vi "PXI_Host_FXP_Read_OldMethod_Benchmark.vi"() -> ()   [LabVIEW 2018]
uses:
  <vilib>/addons/FPGA Advanced Session Resources/LVFPGA Adv Session Resources/OpenByNameSubVI.vi
  <vilib>/rvi/interface/common/dynamic/niFpgaEscapeDelimiterAndNull.vi
  <vilib>/Utility/error.llb/Error Cluster From Error Code.vi
  <vilib>/rvi/errors/niLvFpgaAdjustHostInterfaceError.vi
  <vilib>/FPGAPlugInAG/Dynamic/niLvFpga_Close_Dynamic.vi
  <vilib>/addons/FPGA Advanced Session Resources/LVFPGA Adv Session Resources/OpenByName.xnode
  <vilib>/rvi/interface/nirviReadWriteControl/nirviReadWriteControl.xnode
  <vilib>/rvi/interface/nirviCloseFPGA/nirviCloseFPGA.xnode
  <vilib>/rvi/interface/Simulation/niFpgaSimulationCallBeginRW.vi
  NiFpgaLv.dll
  <vilib>/addons/FPGA Advanced Session Resources/LVFPGA Adv Session Resources/LVFPGAAdvSessionResources.lvlib
panel:
  out "Value out":fxp<+/-,32,16>
  out "error out":errorcluster
  out "Execution time (s)":dbl
  # "Recorded time"
  # "3.37551E-5"
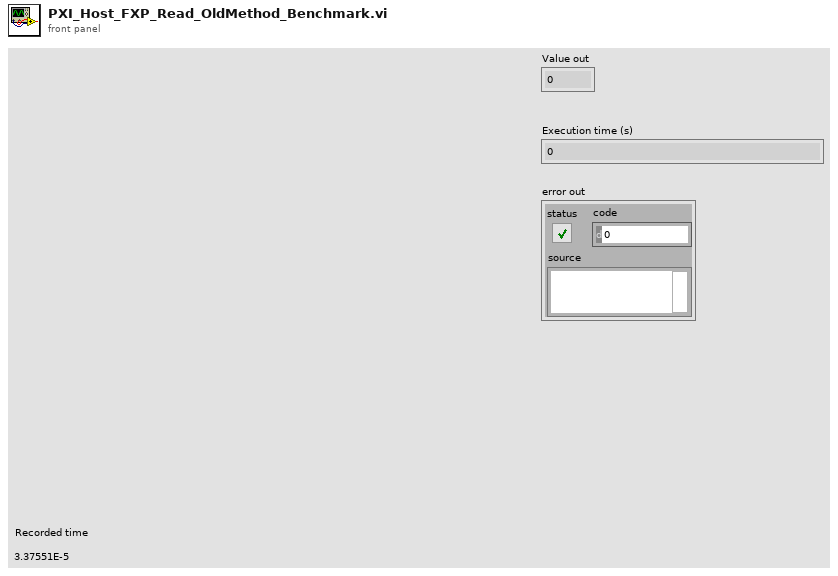
[diagram p1: front panel]
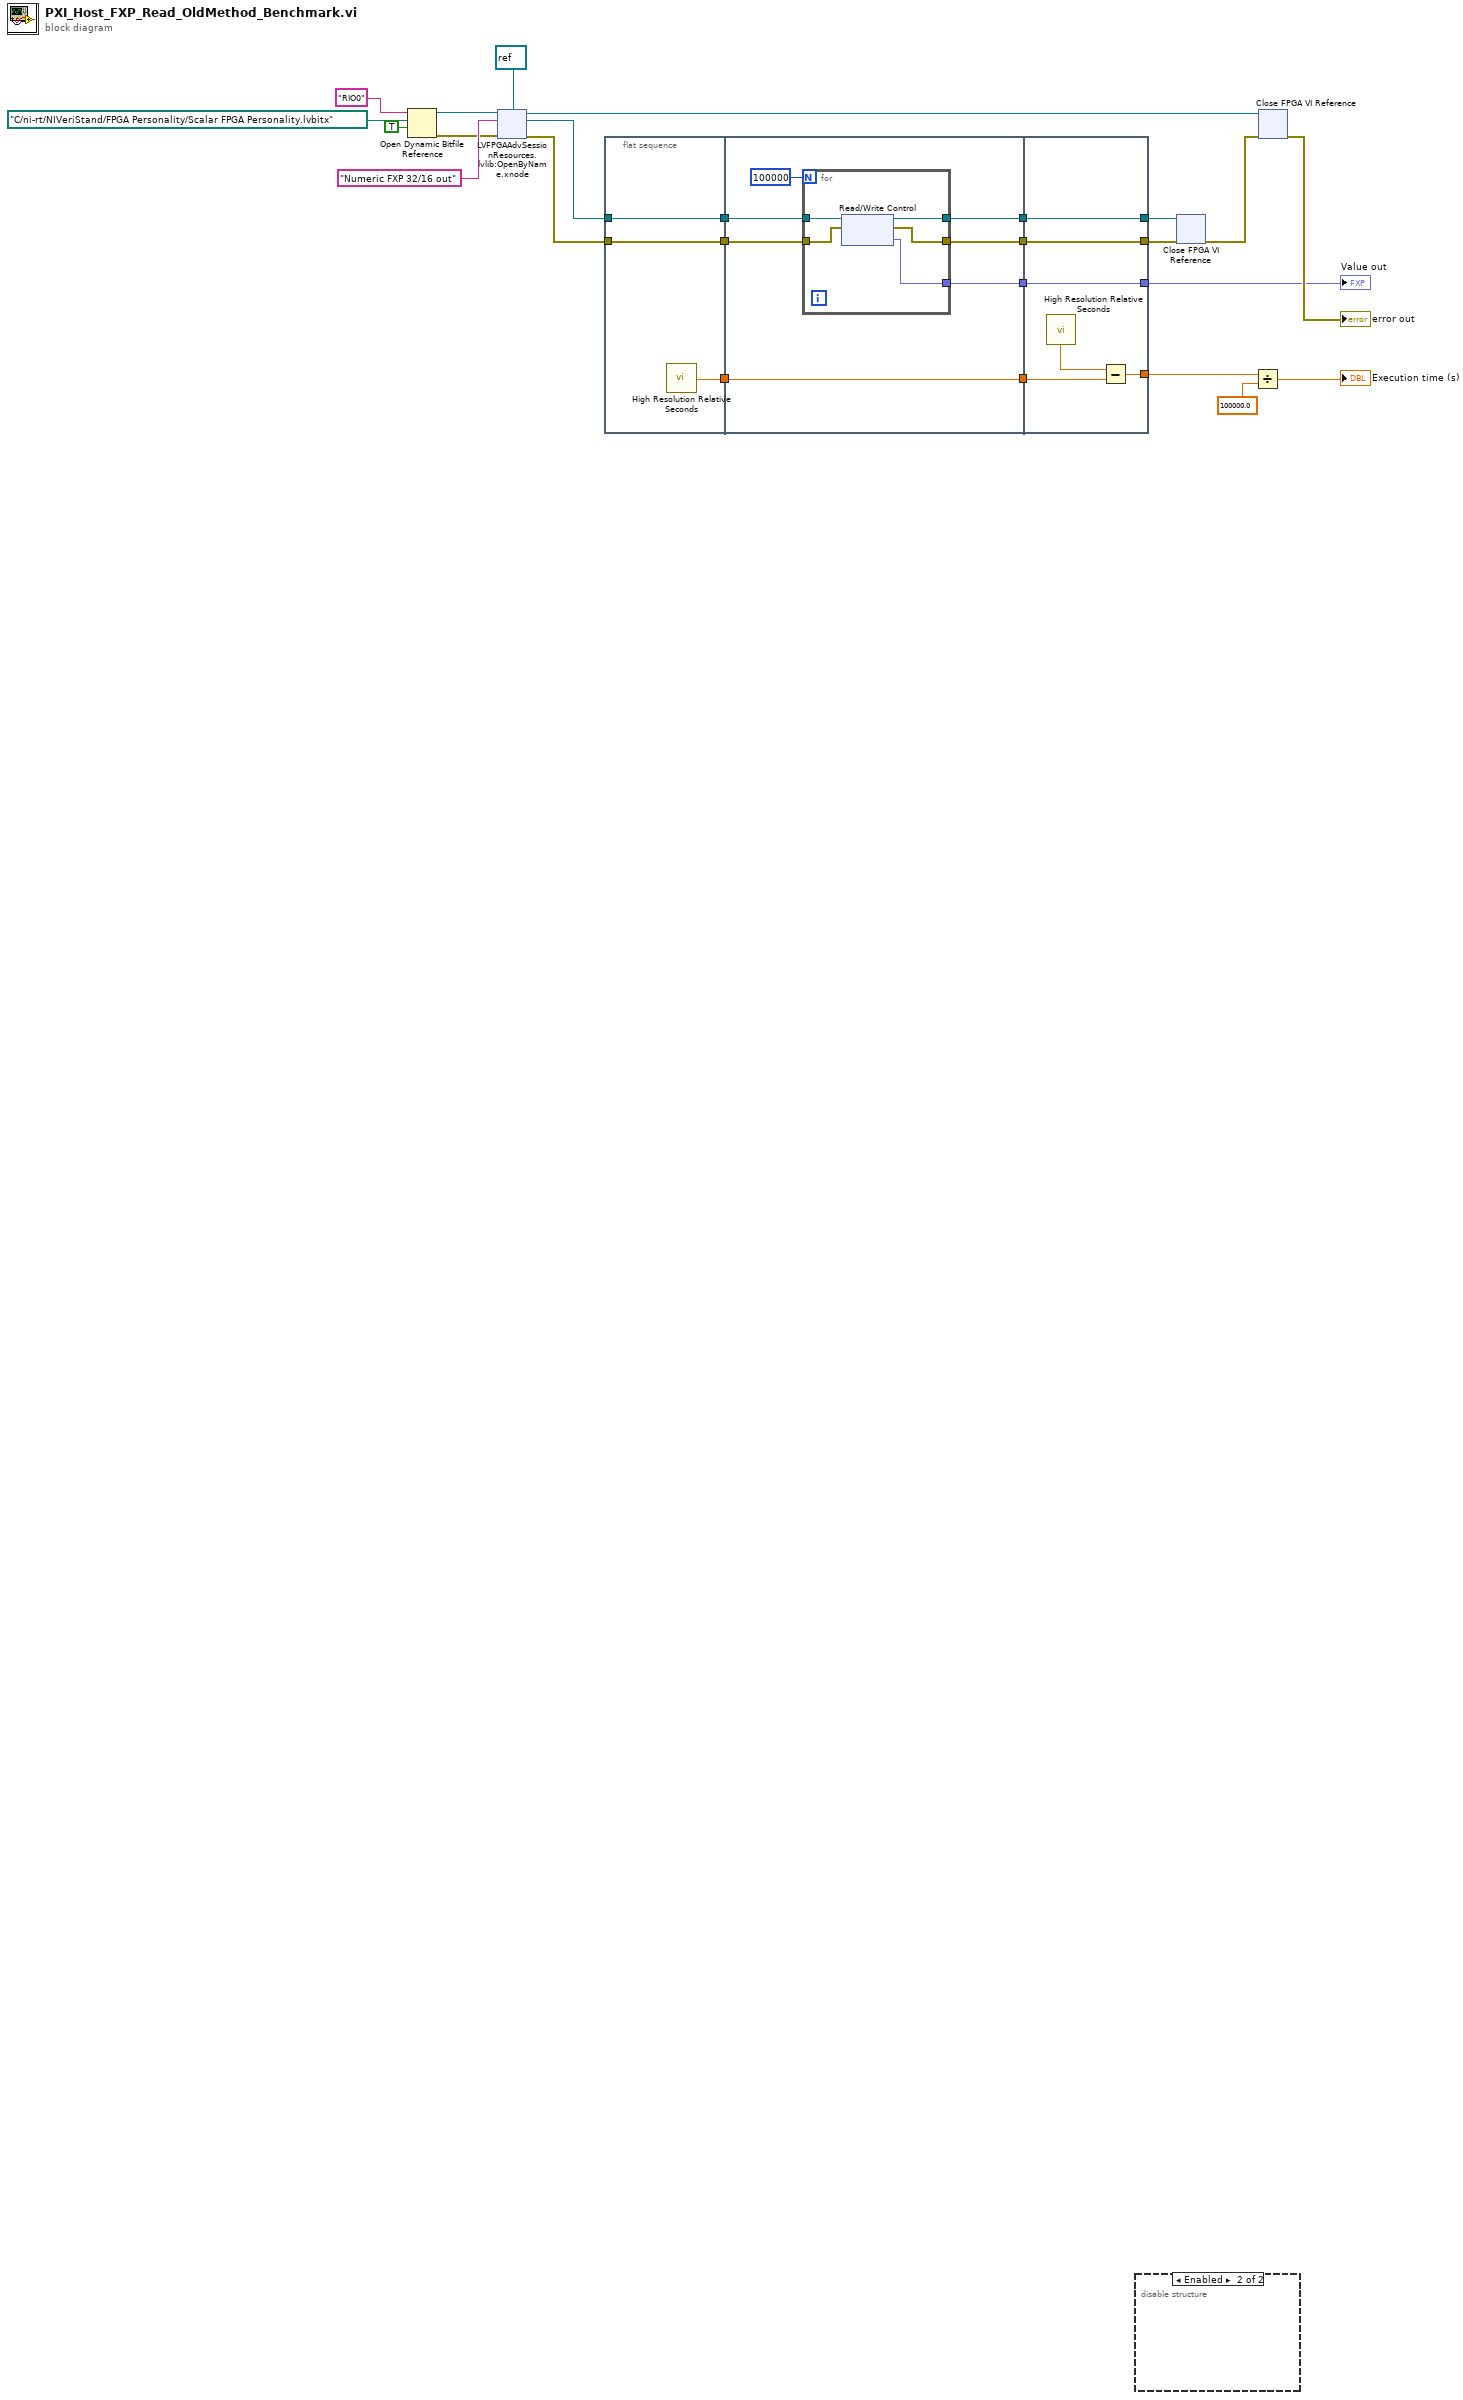
[diagram p0: block diagram]
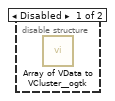
[diagram p2: hidden frame]
diagram:
  n1 = Open Dynamic Bitfile Reference(0:"RIO0" ("Device address"), 1:path "C:/ni-rt/NIVeriStand/FPGA Personality/Scalar FPGA Personality.lvbitx" ("Bitfile path"), 2:TRUE ("Run When Loaded")) -> (5:w13:refnum<k20>, 8:w11:errorcluster)  [unwired: 2 in]
  n2 = xnode "LVFPGAAdvSessionResources.lvlib:OpenByName.xnode"("FPGA VI Reference in"=w13, "Resource name in"="Numeric FXP 32/16 out", "Single resource reference type in"=refnum<k20> refnum ("Type"), "Error in"=w11) -> ("Single resource reference out"=w9:refnum<k20>, "Error out"=w10:errorcluster, "FPGA VI Reference out"=w3:refnum<k20>)
  n3 = flat-sequence {
    tunnel: [w28] -> w24
    tunnel: w9 -> [w27]
    tunnel: [w27] -> w17
    tunnel: [w26] -> w16
    tunnel: w10 -> [w26]
    tunnel: [w34] -> w25
    tunnel: w24 -> [w34]
    tunnel: w17 -> [w33]
    tunnel: w16 -> [w32]
    tunnel: [w31] -> w15
    tunnel: [w30] -> w7
    tunnel: [w29] -> w6
    tunnel: w25 -> [w45]
    tunnel: [w44] -> w23
    tunnel: w15 -> [w43]
    tunnel: [w43] -> w14
    tunnel: [w42] -> w1
    tunnel: w7 -> [w42]
    tunnel: w6 -> [w41]
    tunnel: [w41] -> w5
    frame #0 {
      n4 = call <vilib>:"High Resolution Relative Seconds.vi"() -> ("relative seconds"=w28:dbl)
    }
    frame #1 {
      n5 = for {
        N: 100000 -> [_]
        tunnel: w33 -> [w40]
        tunnel: w32 -> [w39]
        tunnel: [w38] -> w31
        tunnel: [w37] -> w30
        tunnel: [w36] -> w29
        n6 = xnode "Read/Write Control"("FPGA VI Reference In"=w40, "error in"=w39) -> ("FPGA VI Reference Out"=w36:refnum<k20>, "error out"=w38:errorcluster, "Value"=w37:fxp<+/-,32,16>)
      }
    }
    frame #2 {
      n7 = call <vilib>:"High Resolution Relative Seconds.vi"() -> ("relative seconds"=w46:dbl)
      n8 = Subtract(x=w46, y=w45) -> (x-y=w44:dbl)
    }
  }
  n9 = disable-structure shown="Enabled" {
    frame Disabled {
      n10 = call <userlib>:"Array of VData to VCluster__ogtk.vi"() -> ()  [unwired: 10 in, 2 out]
    }
    frame Enabled {
    }
  }
  n11 = xnode "Close FPGA VI Reference"("FPGA VI Reference In"=w5, "error in"=w14) -> ("error out"=w4:errorcluster)
  n12 = Divide(x=w23, y=100000.0) -> (x/y=→"Execution time (s)":dbl)
  n13 = xnode "Close FPGA VI Reference"("FPGA VI Reference In"=w3, "error in"=w4) -> ("error out"=→"error out":errorcluster)
  "Value out" <- w1
